vi "Dxx To Dkm.vi"(8 "error in (no error)":errorcluster, 10 "units":i32, 11 "dXx":dbl) -> (0 "error out":errorcluster, 3 "dkm":dbl)   [LabVIEW 2023, in "POSCONV.lvlib"]
doc: "Converts double input into double kilometres to any of the following units by setting the Units Control:\n\n1. case IN_MI:\n2. case IN_KM:\n3. case IN_M:\n4. case IN_ST:\n5. case IN_DMI:\n\ndouble DxxToDkm(double dXx, int units);"
uses:
  POSCONV.lvlib
  C:/Users/J Gordon/Documents/Rail Tech/TV-HR/02 - Code/Modules/POSCONV/POSCONV.dll
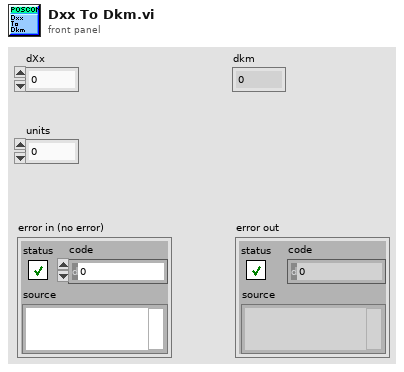
[diagram p1: front panel]
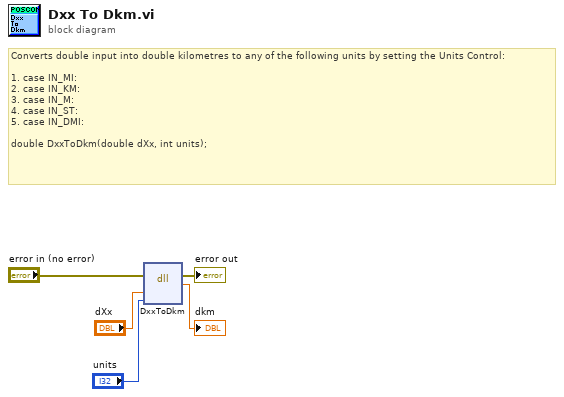
[diagram p0: block diagram]
diagram:
  # "Converts double input into double kilometres to any of the following units by setting the Units Control:\n\n1. case IN_MI:\n2.\tcase IN_KM:\n3.\tcase IN_M:\n4.\tcase IN_ST:\n5.\tcase IN_DMI:\n\ndouble DxxToDkm(double dXx, int units);"
  n1 = dll-call lib="C:/Users/J Gordon/Documents/Rail Tech/TV-HR/02 - Code/Modules/POSCONV/POSCONV.*" fn="DxxToDkm"(error in="error in (no error)", "dXx"="dXx", "units"="units") -> (error out=→"error out":errorcluster, →"dkm":dbl)  [unwired: 4 in, 1 out]
